vi "Write.vi"(8 "error in (no error)":errorcluster, 11 "Channel Manager in":refnum<class "Channel Manager.lvclass">) -> (0 "error out":errorcluster, 3 "Channel Manager out":refnum<class "Channel Manager.lvclass">)   [LabVIEW 2024, in "Embedded TDMS Logger Engine.lvlib" / "Channel Manager.lvclass"]
doc: "Writes to our system channels the current status of our trigger and this iterations error code."
uses:
  Channel Manager.lvclass
  Channel Manager.lvclass/Channel Manager.ctl
  <vilib>/NI/NIVS Inline Async API/_Data Access Engine/Access Type Classes/Write/Write.lvclass/Write.ctl
  <vilib>/NI/NIVS Inline Async API/_Data Access Engine/Data Access Engine/Methods/Write.Data.vi
  <vilib>/NI/NIVS Inline Async API/_Data Access Engine/Access Type Classes/Write/Write.ProcessData.vi
  <vilib>/NI/NIVS Inline Async API/_Data Access Engine/Data Access Engine/Data Access Engine.lvclass
  Embedded TDMS Logger Engine.lvlib
panel:
  out "appended array":dbl[](array[numeric])
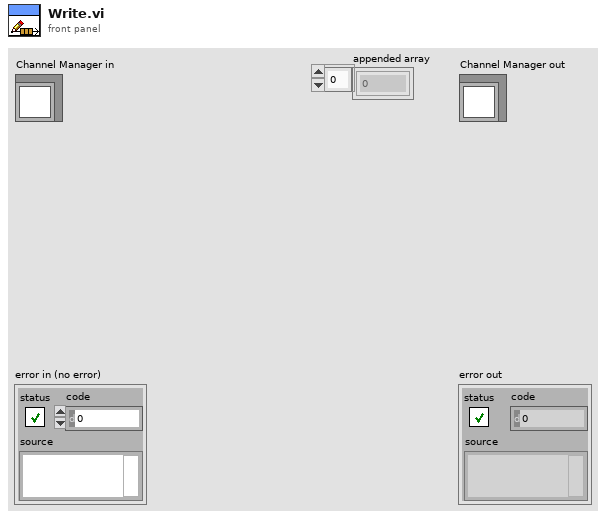
[diagram p1: front panel]
types:
  T1 = typedef "Data Access Engine.lvlib/Data Access Engine.lvclass/Write.DVR.ctl" = refnum<data-value>
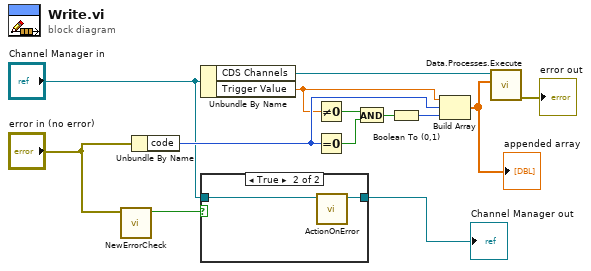
[diagram p0: block diagram]
diagram:
  n1 = call "NewErrorCheck.vi"("error in (no error)"="error in (no error)") -> ("Activate Script?"=w1:bool)  [unwired: 10 in]
  n2 = Unbundle By Name("error in (no error)") -> ("code"=w10:i32)
  n3 = Unbundle By Name("Channel Manager in") -> ("CDS Channels"=w11:T1, "Trigger Value"=w9:dbl)
  n4 = case shown="True" w1 {
    tunnel: "Channel Manager in" -> [w14 w16]
    tunnel: [w14 w15] -> w3
    frame False {
    }
    frame True {
      n5 = call-dynamic "ActionOnError.vi"("Channel Manager in"=w16) -> ("Channel Manager out"=w15:refnum<class "Channel Manager.lvclass">)  [unwired: 9 in, 1 out]
    }
  }
  "Channel Manager out" <- w3
  n6 = Not Equal To 0?(x=w9) -> (x != 0?=w8:bool)
  n7 = Equal To 0?(x=w10) -> (x = 0?=w7:bool)
  n8 = And(x=w8, y=w7) -> (x .and. y?=w6:bool)
  n9 = Boolean To (0,1)(Boolean=w6) -> (0, 1=w5:i16)
  n10 = Build Array(w9, w10, w5) -> (w12:dbl[])
  "appended array" <- w12
  n11 = call-poly <vilib>:"Data.Processes.Execute.vi"("Values"=w12, "Ref"=w11) -> ("error out"=→"error out":errorcluster)  [unwired: 9 in]
